vi "Rotate Buffer.vi"(7 "#bytes per value":i32, 8 "Full?":bool, 9 "Index":i32, 10 "Values":u8[](array[numeric]), 11 "Timestamps":u64[](array[numeric])) -> (1 "empty buffer?":bool, 2 "Values":u8[](array[numeric]), 3 "Timestamps":u64[](array[numeric]))   [LabVIEW 2021, in "Ring Buffer Time Series Data.lvlib"]
uses:
  Ring Buffer Time Series Data.lvlib
  Enforce array size multiple timestamps.vi
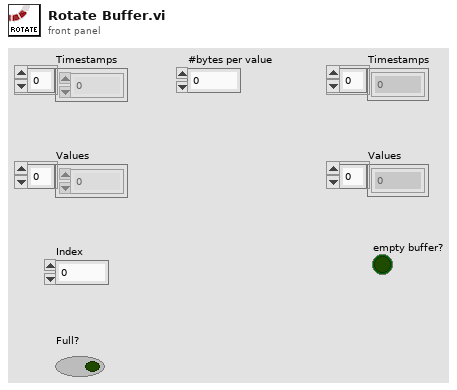
[diagram p1: front panel]
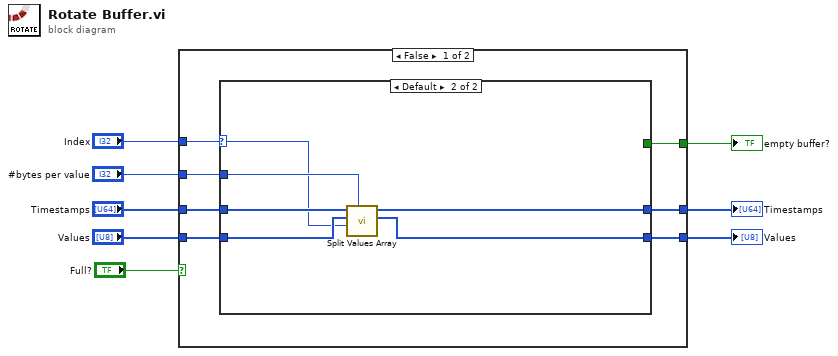
[diagram p0: block diagram]
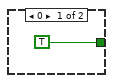
[diagram p2: hidden frame]
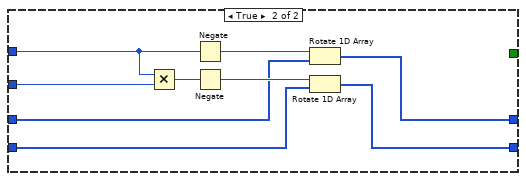
[diagram p3: hidden frame]
diagram:
  n1 = case shown="False" "Full?" {
    tunnel: "Timestamps" -> [w15 w28]
    tunnel: "Values" -> [w14 w27]
    tunnel: [w11 w26] -> w6
    tunnel: [w10 w25] -> w5
    tunnel: "#bytes per value" -> [w13 w24]
    tunnel: "Index" -> [w12 w23]
    tunnel: [w9 _] -> w1
    frame False {
      n2 = case shown="Default" w12 {
        selector: w12 -> [_ w19]
        tunnel: w15 -> [_ w22]
        tunnel: w14 -> [_ w21]
        tunnel: w13 -> [_ w20]
        tunnel: [_ w18] -> w11
        tunnel: [_ w17] -> w10
        tunnel: [TRUE _] -> w9
        frame 0 {
        }
        frame Default {
          n3 = call "Split Values Array.vi"("#bytes per timestamp"=w20, "split index"=w19, "Values"=w21, "Timestamps"=w22) -> ("Values (pre-split)"=w17:u8[], "Timestamps (pre-split)"=w18:u64[])  [unwired: 4 in, 2 out]
        }
      }
    }
    frame True {
      n4 = Multiply(x=w23, y=w24) -> (x*y=w29:i32)
      n5 = Negate(x=w23) -> (-x=w31:i32)
      n6 = Negate(x=w29) -> (-x=w30:i32)
      n7 = Rotate 1D Array(1:w28, 2:w31) -> (0:w26:u64[])
      n8 = Rotate 1D Array(1:w27, 2:w30) -> (0:w25:u8[])
    }
  }
  "Timestamps" <- w6
  "Values" <- w5
  "empty buffer?" <- w1
